vi "Post-Processing VI.vi"() -> ()   [LabVIEW 2014]
uses:
  ATS-VI/ATS_ctl/ExtTrigRange.ctl
  ATS-VI/ATS_ctl/Coupling.ctl
  ATS-VI/ATS_ctl/ExtTrigger.ctl
  ATS-VI/ATS_ctl/TriggerEngine.ctl
  ATS-VI/ATS_ctl/TriggerOperation.ctl
  ATS-VI/ATS_ctl/Trigger.ctl
  ATS-VI/ATS_ctl/Bandwidth.ctl
  ATS-VI/ATS_ctl/Impedance.ctl
  ATS-VI/ATS_ctl/Range.ctl
  ATS-VI/ATS_ctl/InputCtrl.ctl
  ATS-VI/ATS_ctl/ClockEdge.ctl
  ATS-VI/ATS_ctl/ClockRate.ctl
  ATS-VI/ATS_ctl/ClockSource.ctl
  ATS-VI/ATS_ctl/Clock.ctl
  ATS-VI/ATS_ctl/Record.ctl
  ATS-VI/ATS_ctl/ATS_Global.ctl
  Classes/Galvo/Scanning Cluster.ctl
  Classes/Galvo/Galvo.lvclass
  Type Defs/OCT Imaging Parameters Cluster.ctl
  <vilib>/Analysis/NI_AALBase.lvlib
  Type Defs/Imaging Parameters.ctl
  Type Defs/Datalog Format abm.ctl
panel:
  out "No. B-scans":i32=60
  out "system params":T1={"Points Per A-Scan"=0, "A-Scans per B-Scan"=0, "Voltage Range"=4.0, "Card Resolution (bits)"=16}
  in  "Input Parameters":T1={"Points Per A-Scan"=0, "A-Scans per B-Scan"=0, "Voltage Range"=4.0, "Card Resolution (bits)"=16}
  in  "Tab Control":enum32{"Aligned image"}(tab)
  out "Intensity Graph":u8[][](graph)
  in  "Create 3D Data":bool=TRUE
  in  "Max":dbl format="%0.2f"
  in  "Min":dbl format="%0.2f"
  out "Binary File Handle":refnum<file>
  out "En Face":dbl[][](graph)
  out "error out":errorcluster
  out "B-Scan Averaged Across A-Scans":dbl[][](array[numeric])
  in  "En Face Upper Depth":i32=60
  in  "En Face Lower Depth":i32=300
  in  "Cluster":T2={"Imaging Cluster"={"Gain"=6.10352e-05, "Bias"=2.0, "Points Per A-Scan"=-20, "A-Scans per B-Scan"=-20, "Max"=-20.0, "Min"=-20.0}, "OCT Data"=[], "Clock Data"=[]}
  in  "Save B-scans to bmp":bool
  in  "Slide":i32(slide) scale=-1.0..511.0
  in  "Save Image":bool
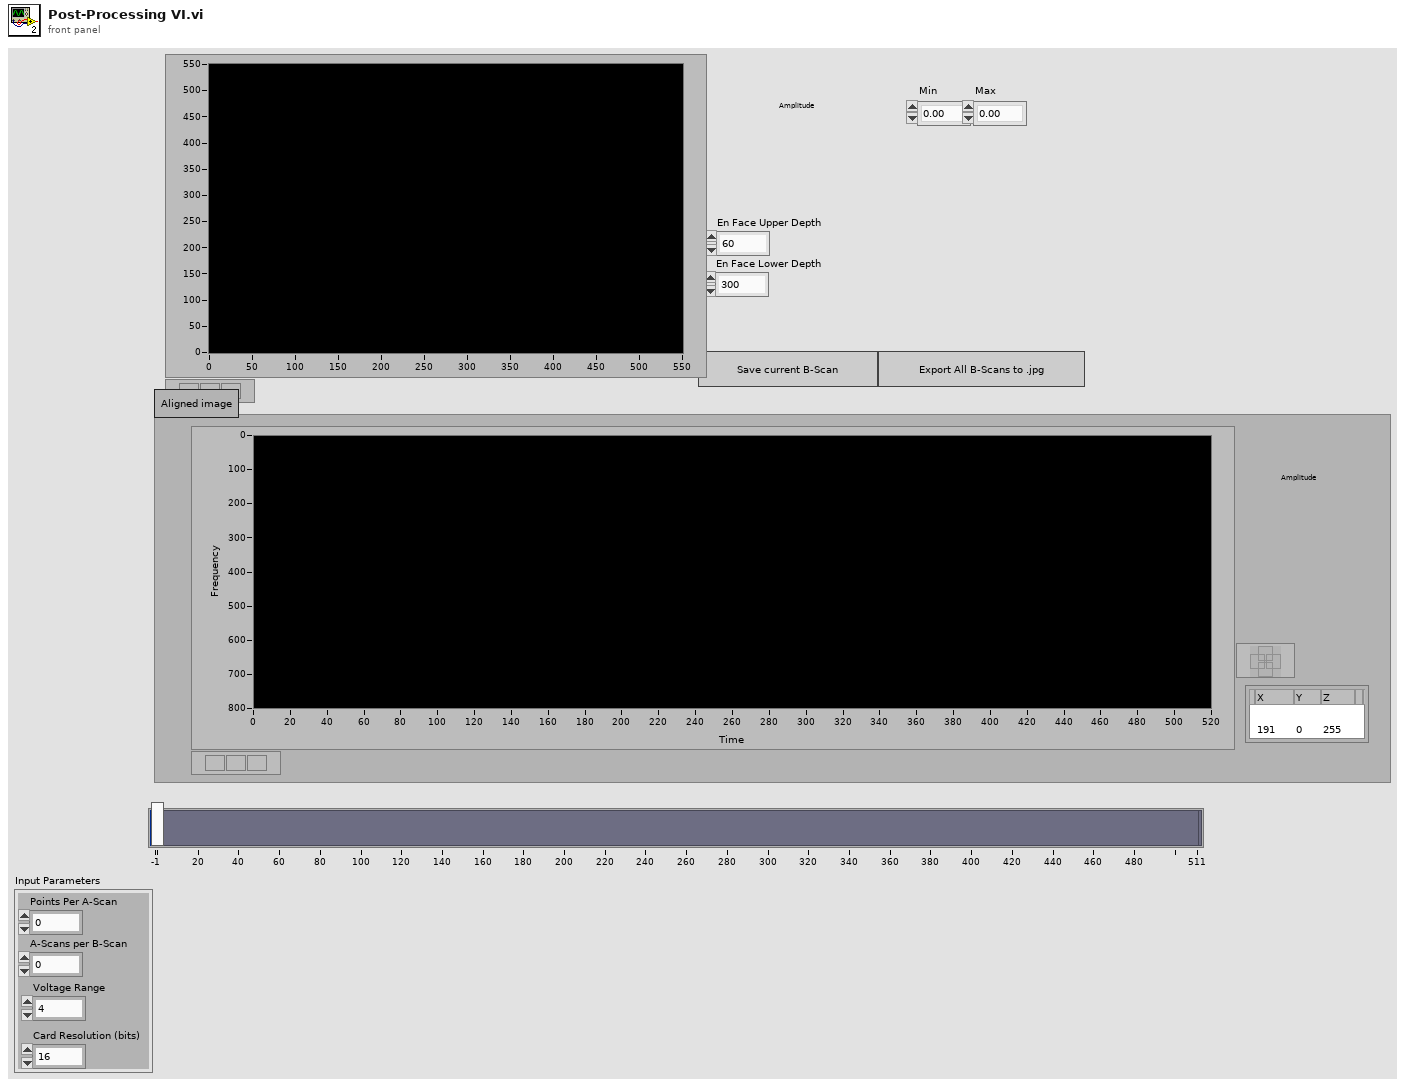
[diagram p1: front panel]
types:
  T1 = typedef "OCT Imaging Parameters Cluster.ctl" = cluster{"Points Per A-Scan":i32, "A-Scans per B-Scan":i32, "Voltage Range":sgl, "Card Resolution (bits)":u16}
  T2 = typedef "Datalog Format abm.ctl" = cluster{"Imaging Cluster":T3, "OCT Data":u16[], "Clock Data":u16[]}
  T3 = typedef "Imaging Parameters.ctl" = cluster{"Gain":sgl, "Bias":sgl, "Points Per A-Scan":i32, "A-Scans per B-Scan":i32, "Max":sgl, "Min":sgl}
  T4 = typedef "Galvo.lvclass/Scanning Cluster.ctl" = cluster{"Fast Axis Offset":sgl, "Slow Axis Offset":sgl, "Slow Axis Amp":sgl, "Fast Axis Amp":sgl, "B-scans (rings)":u32, "A(cluster)/B":u32, "Scan Pattern":enum16{"Raster"}}
  T5 = typedef "ATS_Global.ctl" = cluster{"Record":T6, "Clock":T7, "Input A":T11, "Input B":T11, "Trigger":T16}
  T6 = typedef "Record.ctl" = cluster{"Count":u32, "Presize":u32, "Length":u32}
  T7 = typedef "Clock.ctl" = cluster{"ClckSource":T8, "ClckRate":T9, "ClckEdge":T10, "Decimation":u32}
  T8 = typedef "ClockSource.ctl" = enum16{"Internal", "External", "Medium Ext.", "Slow Ext.", "Ext. AC", "Ext. DC", "Ext. (PLL)"}
  T9 = typedef "ClockRate.ctl" = u32
  T10 = typedef "ClockEdge.ctl" = u16
  T11 = typedef "InputCtrl.ctl" = cluster{"Coupling":T12, "Range":T13, "Impedance":T14, "Bandwidth":T15}
  T12 = typedef "Coupling.ctl" = enum16{"AC", "DC"}
  T13 = typedef "Range.ctl" = u32
  T14 = typedef "Impedance.ctl" = enum16{"1M ohms", "50 ohms"}
  T15 = typedef "Bandwidth.ctl" = enum16{"Full Bandwidth", "Reduce Bandwidth"}
  T16 = typedef "Trigger.ctl" = cluster{"TrigOperation":T17, "Timeout (s)":dbl, "Trig. Delay":u32, "Engine X":T18, "Engine Y":T18, "ExtTrigControl":T19}
  T17 = typedef "TriggerOperation.ctl" = enum16{"Only X", "Only Y", "X or Y", "X and Y", "X xor Y", "X and not Y", "not X and Y"}
  T18 = typedef "TriggerEngine.ctl" = cluster{"Source":enum32{"Chan_A", "Chan_B", "External", "Disable"}, "Slope":enum32{"Positive", "Negative"}, "Level":u32}
  T19 = typedef "ExtTrigger.ctl" = cluster{"Coupling":T12, "Range":T20}
  T20 = typedef "ExtTrigRange.ctl" = enum16{"1 V", "5 V", "TTL"}
  T21 = typedef "imagedata.ctl" = cluster{"image type":i32, "image depth":i32, "image":u8[], "mask":u8[], "colors":u32[], "Rectangle":cluster{"left":i16, "top":i16, "right":i16, "bottom":i16}}
  T22 = cluster{"X Values":dbl[], "Histogram: h(x)":i32[]}
  T23 = typedef "LVRangeTypeDef.ctl" = cluster{"Minimum":dbl, "Maximum":dbl, "Increment":dbl, "Minor Increment":dbl, "Start":dbl}
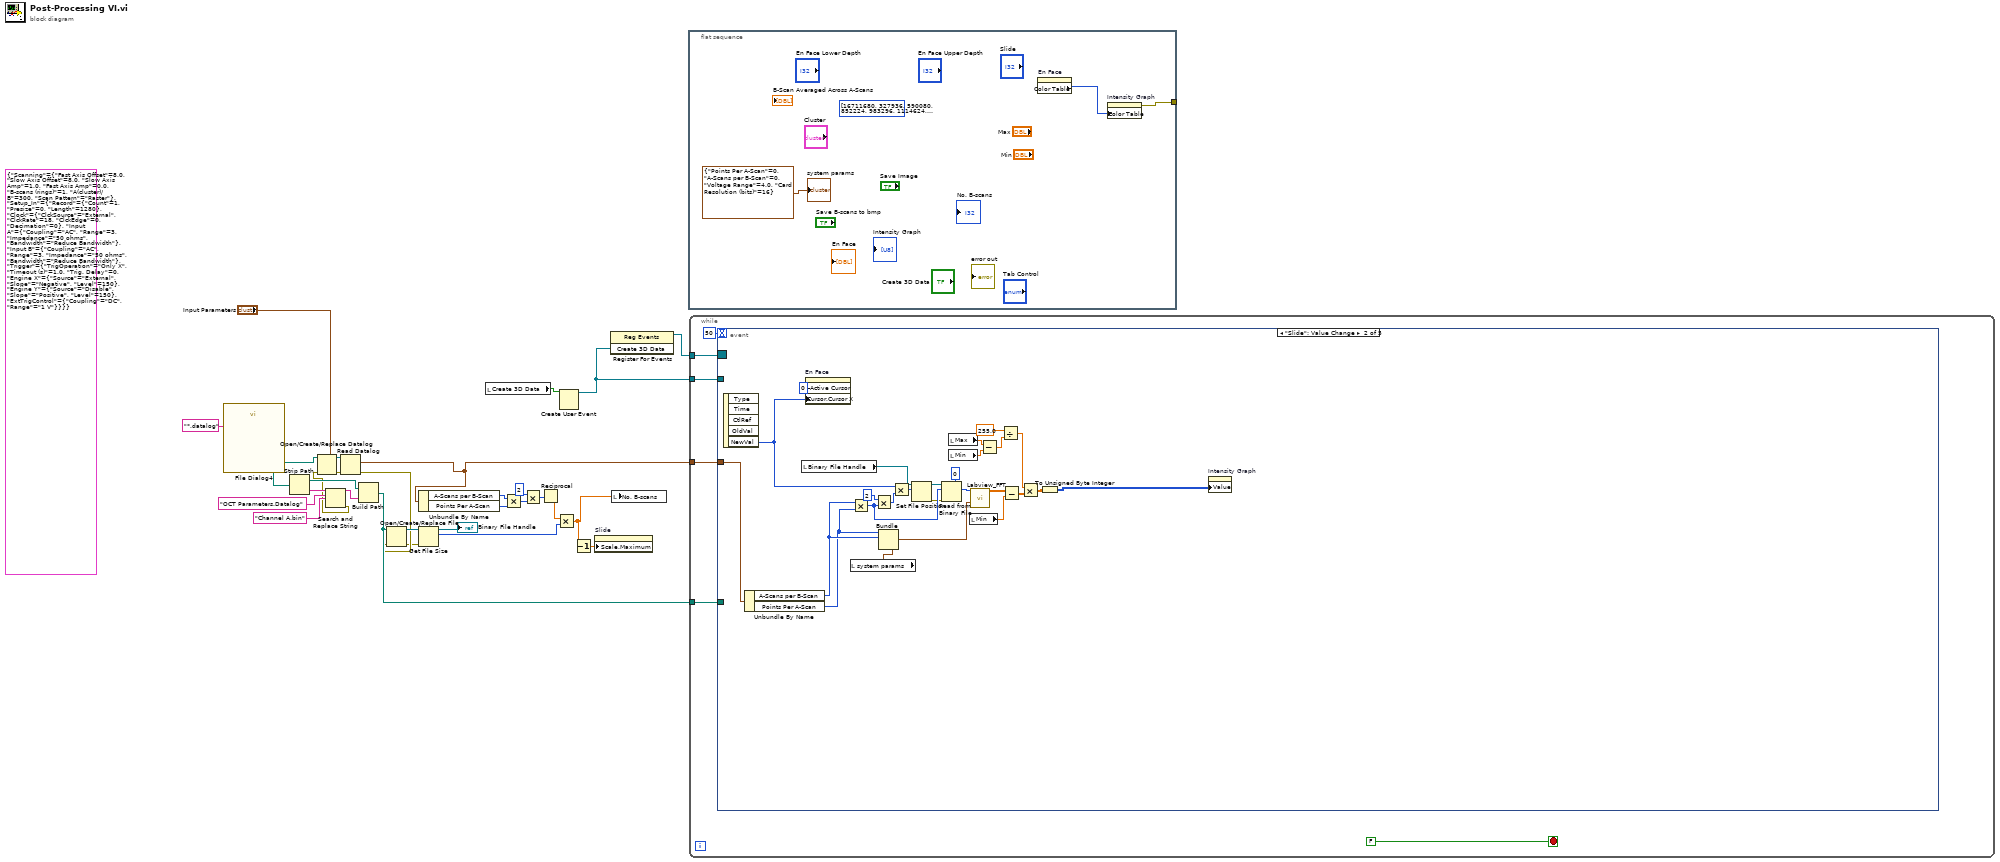
[diagram p0: block diagram]
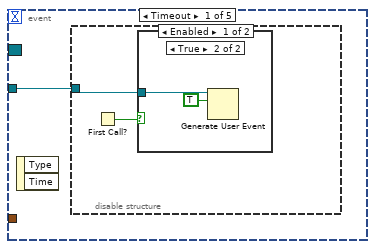
[diagram p2: hidden frame]
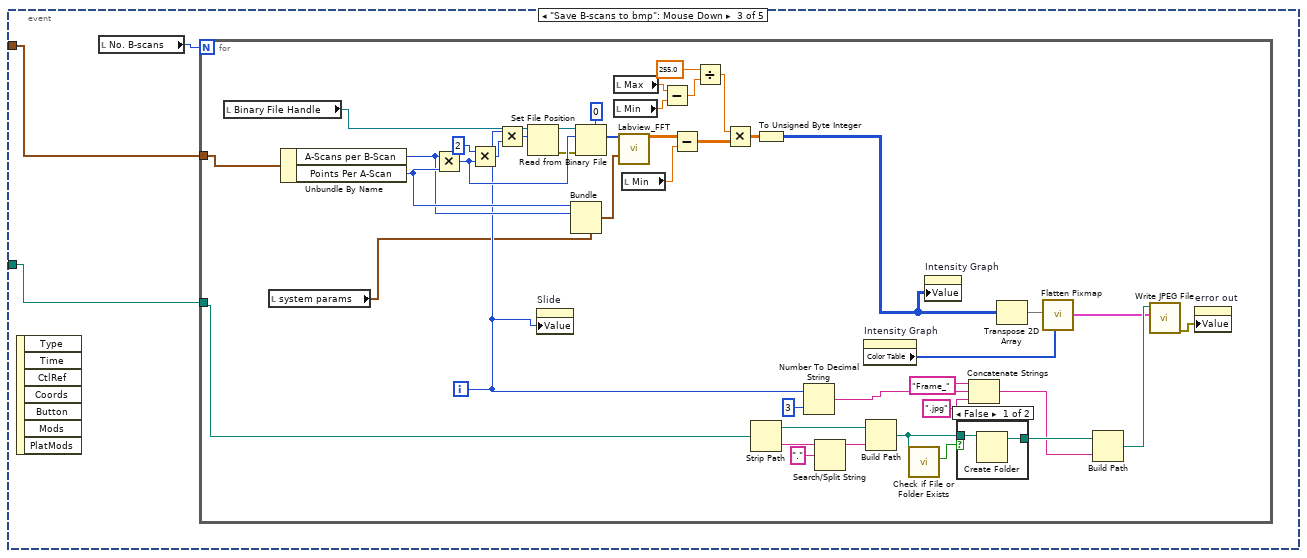
[diagram p5: hidden frame]
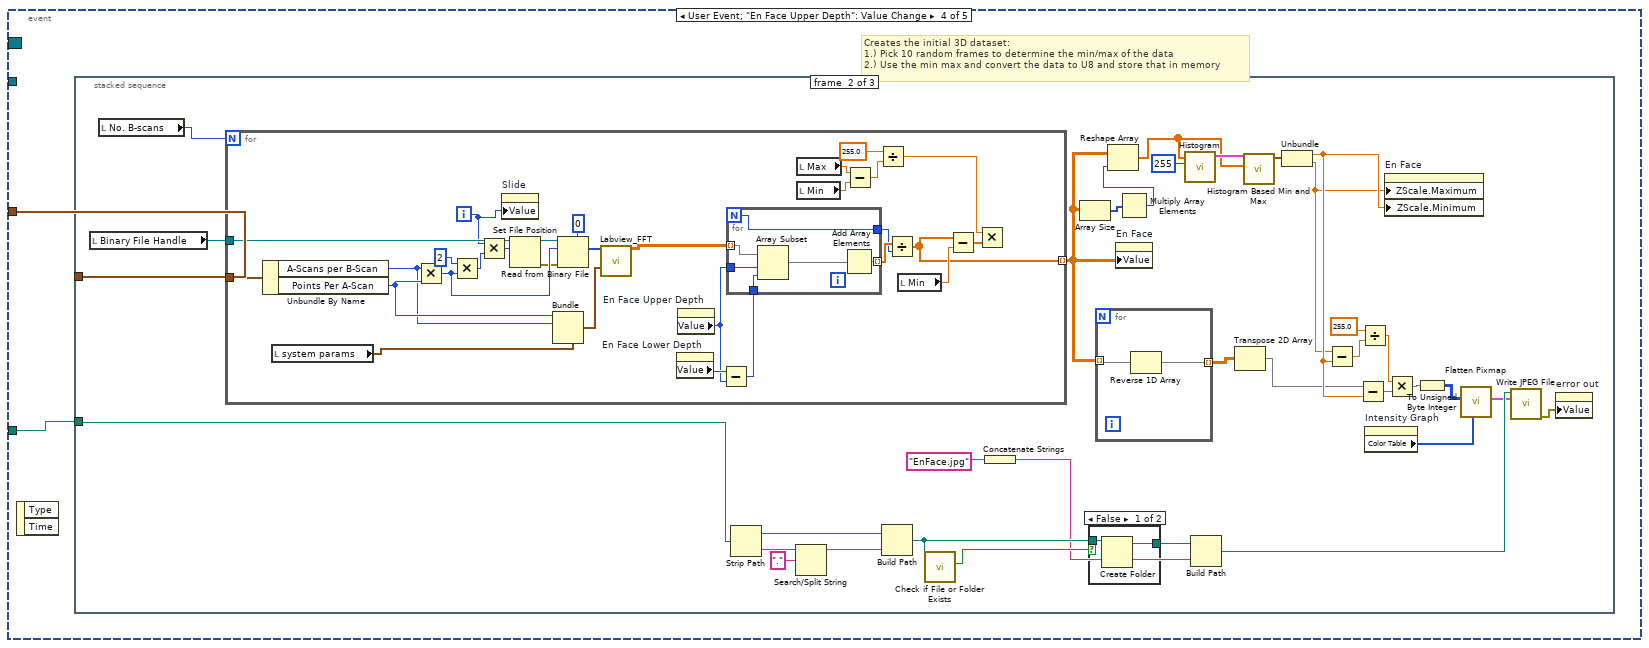
[diagram p7: hidden frame]
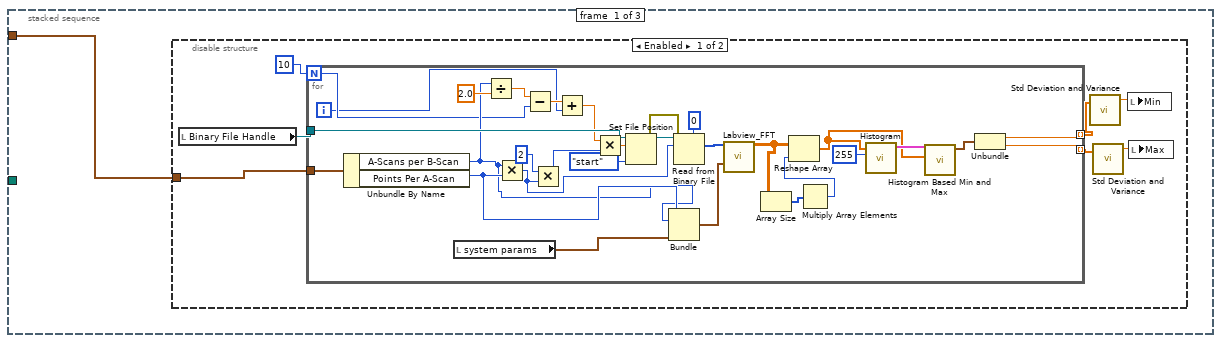
[diagram p8: hidden frame]
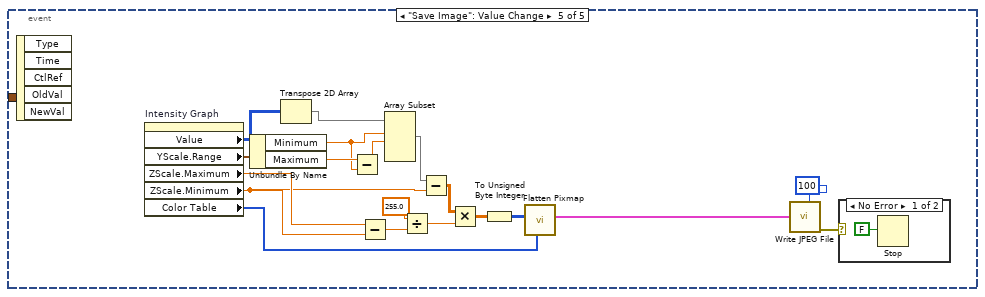
[diagram p12: hidden frame]
diagram:
  (unwired) cluster{"Scanning":T4, "Setup_In":T5} {"Scanning"={"Fast Axis Offset"=8.0, "Slow Axis Offset"=8.0, "Slow Axis Amp"=1.0, "Fast Axis Amp"=0.0, "B-scans (rings)"=1, "A(cluster)/B"=300, "Scan Pattern"=enum."Raster"}, "Setup_In"={"Record"={"Count"=1, "Presize"=0, "Length"=1280}, "Clock"={"ClckSource"=enum."External", "ClckRate"=18, "ClckEdge"=0, "Decimation"=0}, "Input A"={"Coupling"=enum."AC", "Range"=3, "Impedance"=enum."50 ohms", "Bandwidth"=enum."Reduce Bandwidth"}, "Input B"={"Coupling"=enum."AC", "Range"=3, "Impedance"=enum."50 ohms", "Bandwidth"=enum."Reduce Bandwidth"}, "Trigger"={"TrigOperation"=enum."Only X", "Timeout (s)"=1.0, "Trig. Delay"=0, "Engine X"={"Source"=enum."External", "Slope"=enum."Negative", "Level"=150}, "Engine Y"={"Source"=enum."Disable", "Slope"=enum."Positive", "Level"=150}, "ExtTrigControl"={"Coupling"=enum."DC", "Range"=enum."1 V"}}}} ("Sampling Info")
  n1 = call "File Dialog4"("pattern (all files)"="*.datalog") -> ("selected path"=w25:path)  [unwired: 11 in, 3 out]
  n2 = Strip Path(path=w25) -> (stripped path=w21:path, name=w28:string)
  n3 = Search and Replace String(input string=w28, search string="OCT Parameters.Datalog" ("pattern (all files)"), replace string="Channel A.bin" ("pattern (all files)")) -> (result string=w22:string, error out=w6:errorcluster)  [unwired: 5 in, 2 out]
  n4 = Open/Create/Replace Datalog(5:"Input Parameters", 8:w6, 11:w25) -> (0:w23:errorcluster, 3:w24:refnum<k1>)  [unwired: 3 in, 1 out]
  n5 = Read Datalog(4:w23, 7:w24) -> (0:w2:errorcluster, 2:w3:T1)  [unwired: 1 in, 1 out]
  n6 = Build Path(base path=w21, name or relative path=w22) -> (appended path=w12:path)
  n7 = Open/Create/Replace File(file path (use dialog)=w12, error in=w2) -> (refnum out=w20:refnum<file>, error out=w1:errorcluster)  [unwired: 4 in, 1 out]
  n8 = Unbundle By Name(w3) -> ("A-Scans per B-Scan"=w19:i32, "Points Per A-Scan"=w18:i32)
  n9 = Get File Size(file=w20, error in=w1) -> (refnum out=→"Binary File Handle":refnum<file>, size (in bytes)=w14:i64)  [unwired: 1 out]
  n10 = local read "Create 3D Data"() -> (w9:bool)
  n11 = Multiply(x=w19, y=w18) -> (x*y=w17:i32)
  n12 = Multiply(x=u32 2 ("y"), y=w17) -> (x*y=w15:u32)
  n13 = Reciprocal(x=w15) -> (1/x=w13:dbl)
  n14 = Multiply(x=w13, y=w14) -> (x*y=w5:dbl)
  n15 = Create User Event(user event datatype=w9) -> (user event=w8:refnum<user-event>)  [unwired: 1 in, 1 out]
  n16 = Decrement(x=w5) -> (x-1=w4:dbl)
  n17 = property on="Slide" class="Slide (strict)"("Scale.Maximum"=w4) -> ()  [unwired: 2 in, 2 out]
  n18 = register-events(w8) -> (reference out=w11:refnum<event-registration>)  [unwired: 2 in, 1 out]
  n19 = local write "No. B-scans"(w5) -> ()
  n20 = flat-sequence {
    tunnel: [w32] -> _
    frame #0 {
      (unwired) u32[] [16711680, 327936, 590080, 852224, 983296, 1114624, 1180160, 1311232, 1442304, 1573632, 1704704, 1770240, 1901312, 1966848, 2098176, 2163712, 2294784, 2491392, 2557184, 2688256, 2753792, 2884864, 2950656, 3081728, 3147264, 3344129, 3475457, 3540993, 3672321, 3738113, 3869185, 3934977, 4066305, 4197633, 4328961, 4394497, 4460289, 4591617, 4657409, 4788481, 4854273, 4985601, 5116929, 5248257, 5314049, 5379841, 5511169, 5576961, 5708033, 5773825, 5905153, 6036482, 6167810, 6233346, 6299138, 6430466, 6496258, 6562050, 6693634, 6759426, 6890754, 7022082, 7087874, 7153666, 7284994, 7350786, 7482114, 7547906, 7613698, 7745026, 7876354, 8007682, 8073474, 8139522, 8205314, 8336642, 8467970, 8533763, 8599555, 8665347, 8731139, 8862467, 8993795, 9059587, 9125380, 9191428, 9257220, 9388548, 9454340, 9520132, 9585924, 9717253, 9848837, 9914629, 9980165, 10045957, 10177541, 10243334, 10309126, 10375174, 10440966, 10572294, 10703623, 10769416, 10835208, 10901256, 10967049, 11033097, 11033609, 11099401, 11165450, 11231242, 11231754, 11297547, 11363339, 11429131, 11495180, 11495692, 11561740, 11693069, 11758861, 11759373, 11825165, 11891214, 11957006, 12022799, 12023311, 12089103, 12220944, 12286736, 12286736, 12352529, 12418577, 12484370, 12550162, 12615954, 12681747, 12747796, 12813588, 12813845, 12879894, 12945686, 13077015, 13142808, 13143064, 13208856, 13274905, 13340697, 13340953, 13472282, 13538075, 13604379, 13670172, 13735964, 13801757, 13867550, 13933343, 13999392, 13999648, 14065441, 14131234, 14197027, 14197541, 14263334, 14329383, 14395176, 14460969, 14592553, 14658346, 14724139, 14789932, 14790189, 14856238, 14922287, 14988080, 15053873, 15054130, 15119923, 15185972, 15251765, 15317559, 15383353, 15449146, 15449660, 15515454, 15515968, 15516226, 15582021, 15582278, 15582536, 15648587, 15648844, 15714639, 15714897, 15715155, 15780949, 15781463, 15847256, 15847770, 15848028, 15913823, 15914081, 15979875, 15980133, 15980391, 16046441, 16046444, 16046703, 16046705, 16112500, 16113015, 16113274, 16113277, 16179072, 16179330, 16179588, 16245384, 16245387, 16245389, 16245648, 16311443, 16376982, 16377241, 16377499, 16443294, 16443553, 16443555, 16443815, 16509866, 16510124, 16510127, 16575923, 16575924, 16576182, 16576441, 16576443, 16576702, 16576705, 16576963, 16577222, 16577224, 16577482, 16577485, 16577743, 16577745, 16578004, 16578262, 16578264, 16578523, 16578782, 16579040, 16579299, 16579301, 16579303, 16579562, 16579821] ("Color Table")
      n21 = property on="En Face" class="IntGraph (strict)"() -> ("Color Table"=w30:u32[])  [unwired: 2 in, 2 out]
      n22 = property on="Intensity Graph" class="IntGraph (strict)"("Color Table"=w30) -> (error out=w32:errorcluster)  [unwired: 2 in, 1 out]
      "system params" <- T1 {"Points Per A-Scan"=0, "A-Scans per B-Scan"=0, "Voltage Range"=4.0, "Card Resolution (bits)"=16} ("Input Parameters")
    }
  }
  n23 = while {
    tunnel: w3 -> [w36]
    tunnel: w12 -> [w35]
    tunnel: w11 -> [w34]
    tunnel: w8 -> [w33]
    stop <- FALSE stop-if-true
    n24 = event shown="[1] \"Slide\": Value Change" {
      selector: w34 -> [_ _ _ _ _]
      dyn-events: _ -> [_ _ _ _ _]
      timeout: 50 -> [_ _ _ _ _]
      tunnel: w36 -> [_ w68 w72 w120 _]
      tunnel: w35 -> [_ _ w71 w119 _]
      tunnel: w33 -> [w39 _ _ _ _]
      event Timeout {
        n25 = event-data() -> ()  [unwired: 1 in, 2 out]
        n26 = disable-structure shown="Enabled" {
          disable-tunnel: w39 -> [w40 _]
          frame Enabled {
            n27 = First Call?() -> (First Call?: T/F=w41:bool)
            n28 = case shown="True" w41 {
              tunnel: w40 -> [_ w43]
              frame False {
              }
              frame True {
                n29 = Generate User Event(user event=w43, event data cluster=TRUE ("event data")) -> ()  [unwired: 2 in, 2 out]
              }
            }
          }
          frame Disabled {
          }
        }
      }
      event "Slide": Value Change {
        n30 = event-data() -> ("NewVal"=w57:i32)  [unwired: 1 in, 4 out]
        n31 = Unbundle By Name(w68) -> ("A-Scans per B-Scan"=w58:i32, "Points Per A-Scan"=w44:i32)
        n32 = local read "Binary File Handle"() -> (w48:refnum<file>)
        n33 = property on="En Face" class="IntGraph (strict)"("Active Cursor"=u32 0, "Cursor.Cursor X"=w57) -> ()  [unwired: 2 in, 2 out]
        n34 = local read "system params"() -> (w47:T1)
        n35 = Multiply(x=w58, y=w44) -> (x*y=w61:i32)
        n36 = Multiply(x=u32 2 ("y"), y=w61) -> (x*y=w63:u32)
        n37 = Bundle(cluster=w47, "Points Per A-Scan"=w44, "A-Scans per B-Scan"=w58) -> (w59:T1)  [unwired: 2 in]
        n38 = Multiply(x=w57, y=w63) -> (x*y=w65:u32)
        n39 = Set File Position(offset (in bytes) (0)=w65, refnum=w48) -> (refnum out=w66:refnum<file>, error out=w60:errorcluster)  [unwired: 2 in]
        n40 = Read from Binary File(5:u16 0 ("width (-)"), 8:w60, 10:w61, 11:w66) -> (2:w64:u16[])  [unwired: 2 in, 3 out]
        n41 = local read "Max"() -> (w54:dbl)
        n42 = local read "Min"() -> (w53:dbl)
        n43 = local read "Min"() -> (w56:dbl)
        n44 = call "Labview_FFT.vi"("Channel A"=w64, "Input Parameters"=w59) -> ("Int B-Scan Channel A"=w46:sgl[][])  [unwired: 12 in, 1 out]
        n45 = Subtract(x=w54, y=w53) -> (x-y=w52:dbl)
        n46 = Divide(x=255.0, y=w52) -> (x/y=w50:dbl)
        n47 = Subtract(x=w46, y=w56) -> (x-y=w51:dbl[][])
        n48 = Multiply(x=w50, y=w51) -> (x*y=w49:dbl[][])
        n49 = To Unsigned Byte Integer(number=w49) -> (unsigned 8bit integer=w45:u8[][])
        n50 = property on="Intensity Graph" class="IntGraph (strict)"("Value"=w45) -> ()  [unwired: 2 in, 2 out]
      }
      event "Save B-scans to bmp": Mouse Down {
        n51 = event-data() -> ()  [unwired: 1 in, 7 out]
        n52 = local read "No. B-scans"() -> (w70:i32)
        n53 = for {
          N: w70 -> [_]
          tunnel: w72 -> [w78]
          tunnel: w71 -> [w100]
          i -> [w75]
          n54 = local read "Binary File Handle"() -> (w77:refnum<file>)
          n55 = local read "system params"() -> (w74:T1)
          n56 = Unbundle By Name(w78) -> ("A-Scans per B-Scan"=w79:i32, "Points Per A-Scan"=w80:i32)
          n57 = Multiply(x=w79, y=w80) -> (x*y=w92:i32)
          n58 = Multiply(x=u32 2 ("y"), y=w92) -> (x*y=w94:u32)
          n59 = Multiply(x=w75, y=w94) -> (x*y=w96:u32)
          n60 = Set File Position(offset (in bytes) (0)=w96, refnum=w77) -> (refnum out=w97:refnum<file>, error out=w91:errorcluster)  [unwired: 2 in]
          n61 = property on="Slide" class="Slide (strict)"("Value"=w75) -> ()  [unwired: 2 in, 2 out]
          n62 = Bundle(cluster=w74, "Points Per A-Scan"=w80, "A-Scans per B-Scan"=w79) -> (w82:T1)  [unwired: 2 in]
          n63 = Read from Binary File(5:u16 0 ("width (-)"), 8:w91, 10:w92, 11:w97) -> (2:w95:u16[])  [unwired: 2 in, 3 out]
          n64 = local read "Max"() -> (w88:dbl)
          n65 = local read "Min"() -> (w87:dbl)
          n66 = call "Labview_FFT.vi"("Channel A"=w95, "Input Parameters"=w82) -> ("Int B-Scan Channel A"=w81:sgl[][])  [unwired: 12 in, 1 out]
          n67 = local read "Min"() -> (w90:dbl)
          n68 = Subtract(x=w88, y=w87) -> (x-y=w86:dbl)
          n69 = Subtract(x=w81, y=w90) -> (x-y=w85:dbl[][])
          n70 = Divide(x=255.0, y=w86) -> (x/y=w84:dbl)
          n71 = Multiply(x=w84, y=w85) -> (x*y=w83:dbl[][])
          n72 = Strip Path(path=w100) -> (stripped path=w111:path, name=w113:string)
          n73 = To Unsigned Byte Integer(number=w83) -> (unsigned 8bit integer=w76:u8[][])
          n74 = Number To Decimal String(number=w75, width (-)=i16 3) -> (decimal integer string=w109:string)
          n75 = Search/Split String(string=w113, search string/char (-)=".") -> (substring before match=w112:string)  [unwired: 1 in, 2 out]
          n76 = property on="Intensity Graph" class="IntGraph (strict)"() -> ("Color Table"=w115:u32[])  [unwired: 2 in, 2 out]
          n77 = Build Path(base path=w111, name or relative path=w112) -> (appended path=w103:path)
          n78 = call <vilib>:"Check if File or Folder Exists.vi"("path"=w103) -> ("file or folder exists?"=w102:bool)  [unwired: 8 in, 2 out]
          n79 = property on="Intensity Graph" class="IntGraph (strict)"("Value"=w76) -> ()  [unwired: 2 in, 2 out]
          n80 = case shown="False" w102 {
            tunnel: [w117 w118] -> w106
            tunnel: w103 -> [w116 w118]
            frame False {
              n81 = Create Folder(path (use dialog)=w116) -> (created path=w117:path)  [unwired: 2 in, 2 out]
            }
            frame True {
            }
          }
          n82 = Concatenate Strings("Frame_" ("string"), w109, ".jpg" ("string")) -> (w105:string)
          n83 = Transpose 2D Array(2D array=w76) -> (transposed array=w104:u8[][])
          n84 = call <vilib>:"Flatten Pixmap.vi"("colors"=w115, "8-bit pixmap"=w104) -> ("image data"=w73:T21)  [unwired: 9 in]
          n85 = Build Path(base path=w106, name or relative path=w105) -> (appended path=w101:path)
          n86 = call <vilib>:"Write JPEG File.vi"("image data"=w73, "path to JPEG file"=w101) -> ("error out"=w99:errorcluster)  [unwired: 8 in, 1 out]
          n87 = property on="error out" class="Clust (strict)"("Value"=w99) -> ()  [unwired: 2 in, 2 out]
        }
      }
      event User Event; "En Face Upper Depth": Value Change {
        # "Creates the initial 3D dataset:\n1.) Pick 10 random frames to determine the min/max of the data\n2.) Use the min max and convert the data to U8 and store that in memory"
        n88 = event-data() -> ()  [unwired: 1 in, 2 out]
        n89 = stacked-sequence {
          tunnel: w120 -> [w121 w191 _]
          tunnel: w119 -> [_ w177 _]
          frame #0 {
            n90 = disable-structure shown="Enabled" {
              disable-tunnel: w121 -> [w126 _]
              frame Enabled {
                n91 = local read "Binary File Handle"() -> (w128:refnum<file>)
                n92 = for {
                  N: 10 -> [w137]
                  tunnel: w126 -> [w154]
                  tunnel: w128 -> [w153]
                  tunnel: [w142] -> w125 mode=indexing
                  tunnel: [w141] -> w124 mode=indexing
                  i -> [w135]
                  n93 = Unbundle By Name(w154) -> ("A-Scans per B-Scan"=w139:i32, "Points Per A-Scan"=w148:i32)
                  n94 = local read "system params"() -> (w147:T1)
                  n95 = Divide(x=w139, y=2.0) -> (x/y=w138:dbl)
                  n96 = Multiply(x=w139, y=w148) -> (x*y=w133:i32)
                  n97 = Subtract(x=w138, y=w137) -> (x-y=w136:dbl)
                  n98 = Multiply(x=u32 2 ("y"), y=w133) -> (x*y=w152:u32)
                  n99 = Add(x=w136, y=w135) -> (x+y=w134:dbl)
                  n100 = Multiply(x=w134, y=w152) -> (x*y=w156:dbl)
                  n101 = Set File Position(offset (in bytes) (0)=w156, refnum=w153, from (0:start)=enum16{"start", "end", "current"}."start") -> (refnum out=w157:refnum<file>, error out=w150:errorcluster)  [unwired: 1 in]
                  n102 = Bundle(cluster=w147, "Points Per A-Scan"=w148, "A-Scans per B-Scan"=w139) -> (w149:T1)  [unwired: 2 in]
                  n103 = Read from Binary File(5:u16 0 ("width (-)"), 8:w150, 10:w133, 11:w157) -> (2:w155:u16[])  [unwired: 2 in, 3 out]
                  n104 = call "Labview_FFT.vi"("Channel A"=w155, "Input Parameters"=w149) -> ("Int B-Scan Channel A"=w132:sgl[][])  [unwired: 12 in, 1 out]
                  n105 = Array Size(array=w132) -> (size(s)=w131:i32[])
                  n106 = Multiply Array Elements(1:w131) -> (0:w130:i32)
                  n107 = Reshape Array(w132, w130) -> (w144:sgl[])
                  n108 = call <vilib>:"Histogram.vi"("intervals"=255, "X"=w144) -> ("Histogram Graph"=w145:T22)  [unwired: 6 in, 3 out]
                  n109 = call "Histogram Based Min and Max.vi"("Data to Histogram"=w144, "Histogram Graph"=w145) -> ("Histogram Properties"=w143:cluster{"Min":sgl, "Max":sgl})  [unwired: 9 in]
                  n110 = Unbundle(w143) -> ("Min"=w142:sgl, "Max"=w141:sgl)
                }
                n111 = call <vilib>:"Std Deviation and Variance.vi"("X"=w125) -> ("mean"=w123:dbl)  [unwired: 1 in, 2 out]
                n112 = call <vilib>:"Std Deviation and Variance.vi"("X"=w124) -> ("mean"=w122:dbl)  [unwired: 1 in, 2 out]
                n113 = local write "Min"(w123) -> ()
                n114 = local write "Max"(w122) -> ()
              }
              frame Disabled {
              }
            }
          }
          frame #1 {
            n115 = local read "Binary File Handle"() -> (w192:refnum<file>)
            n116 = local read "No. B-scans"() -> (w176:i32)
            n117 = for {
              N: w176 -> [_]
              tunnel: w191 -> [w222]
              tunnel: w192 -> [w221]
              tunnel: [w198] -> w161 mode=indexing
              i -> [w209]
              n118 = Unbundle By Name(w222) -> ("A-Scans per B-Scan"=w214:i32, "Points Per A-Scan"=w215:i32)
              n119 = local read "system params"() -> (w210:T1)
              n120 = Multiply(x=w214, y=w215) -> (x*y=w218:i32)
              n121 = Multiply(x=u32 2 ("y"), y=w218) -> (x*y=w220:u32)
              n122 = Multiply(x=w209, y=w220) -> (x*y=w224:u32)
              n123 = property on="Slide" class="Slide (strict)"("Value"=w209) -> ()  [unwired: 2 in, 2 out]
              n124 = Set File Position(offset (in bytes) (0)=w224, refnum=w221) -> (refnum out=w225:refnum<file>, error out=w217:errorcluster)  [unwired: 2 in]
              n125 = Bundle(cluster=w210, "Points Per A-Scan"=w215, "A-Scans per B-Scan"=w214) -> (w216:T1)  [unwired: 2 in]
              n126 = Read from Binary File(5:u16 0 ("width (-)"), 8:w217, 10:w218, 11:w225) -> (2:w223:u16[])  [unwired: 2 in, 3 out]
              n127 = call "Labview_FFT.vi"("Channel A"=w223, "Input Parameters"=w216) -> ("Int B-Scan Channel A"=w208:sgl[][])  [unwired: 12 in, 1 out]
              n128 = property on="En Face Lower Depth" class="DigNum (strict)"() -> ("Value"=w213:i32)  [unwired: 2 in, 2 out]
              n129 = property on="En Face Upper Depth" class="DigNum (strict)"() -> ("Value"=w212:i32)  [unwired: 2 in, 2 out]
              n130 = Subtract(x=w213, y=w212) -> (x-y=w211:i32)
              n131 = for {
                N -> [w230]
                tunnel: w212 -> [w232]
                tunnel: [w231] -> w207 mode=indexing
                tunnel: [w230] -> w206
                tunnel: w211 -> [w229]
                tunnel: w208 -> [w227] mode=indexing
                n132 = Array Subset(array=w227, index=w232, length=w229) -> (w228:sgl[])
                n133 = Add Array Elements(numeric array=w228) -> (sum=w231:sgl)
              }
              n134 = local read "Max"() -> (w204:dbl)
              n135 = local read "Min"() -> (w203:dbl)
              n136 = Subtract(x=w204, y=w203) -> (x-y=w202:dbl)
              n137 = Divide(x=255.0, y=w202) -> (x/y=w199:dbl)
              n138 = Divide(x=w207, y=w206) -> (x/y=w198:sgl[])
              n139 = local read "Min"() -> (w200:dbl)
              n140 = Subtract(x=w198, y=w200) -> (x-y=w201:dbl[])
              n141 = Multiply(x=w199, y=w201) -> ()  [unwired: 1 out]
            }
            n142 = Strip Path(path=w177) -> (stripped path=w182:path, name=w180:string)
            n143 = Search/Split String(string=w180, search string/char (-)=".") -> (substring before match=w181:string)  [unwired: 1 in, 2 out]
            n144 = Build Path(base path=w182, name or relative path=w181) -> (appended path=w186:path)
            n145 = call <vilib>:"Check if File or Folder Exists.vi"("path"=w186) -> ("file or folder exists?"=w187:bool)  [unwired: 8 in, 2 out]
            n146 = Concatenate Strings("EnFace.jpg" ("string")) -> (w185:string)
            n147 = Array Size(array=w161) -> (size(s)=w171:i32[])
            n148 = case shown="False" w187 {
              tunnel: [w196 w197] -> w184
              tunnel: w186 -> [w195 w197]
              frame False {
                n149 = Create Folder(path (use dialog)=w195) -> (created path=w196:path)  [unwired: 2 in, 2 out]
              }
              frame True {
              }
            }
            n150 = for {
              tunnel: w161 -> [w194] mode=indexing
              tunnel: [w193] -> w160 mode=indexing
              n151 = Reverse 1D Array(array=w194) -> (reversed array=w193:sgl[])
            }
            n152 = property on="En Face" class="IntGraph (strict)"("Value"=w161) -> ()  [unwired: 2 in, 2 out]
            n153 = Multiply Array Elements(1:w171) -> (0:w170:i32)
            n154 = Reshape Array(w161, w170) -> (w173:sgl[])
            n155 = call <vilib>:"Histogram.vi"("intervals"=255, "X"=w173) -> ("Histogram Graph"=w174:T22)  [unwired: 6 in, 3 out]
            n156 = Build Path(base path=w184, name or relative path=w185) -> (appended path=w189:path)
            n157 = Transpose 2D Array(2D array=w160) -> (transposed array=w159:sgl[][])
            n158 = call "Histogram Based Min and Max.vi"("Data to Histogram"=w173, "Histogram Graph"=w174) -> ("Histogram Properties"=w172:cluster{"Min":sgl, "Max":sgl})  [unwired: 9 in]
            n159 = Unbundle(w172) -> ("Min"=w163:sgl, "Max"=w162:sgl)
            n160 = Subtract(x=w162, y=w163) -> (x-y=w169:sgl)
            n161 = Subtract(x=w159, y=w163) -> (x-y=w168:sgl[][])
            n162 = Divide(x=sgl 255.0, y=w169) -> (x/y=w167:sgl)
            n163 = property on="Intensity Graph" class="IntGraph (strict)"() -> ("Color Table"=w178:u32[])  [unwired: 2 in, 2 out]
            n164 = property on="En Face" class="IntGraph (strict)"("ZScale.Maximum"=w162, "ZScale.Minimum"=w163) -> ()  [unwired: 2 in, 2 out]
            n165 = Multiply(x=w167, y=w168) -> (x*y=w166:sgl[][])
            n166 = To Unsigned Byte Integer(number=w166) -> (unsigned 8bit integer=w164:u8[][])
            n167 = call <vilib>:"Flatten Pixmap.vi"("colors"=w178, "8-bit pixmap"=w164) -> ("image data"=w188:T21)  [unwired: 9 in]
            n168 = call <vilib>:"Write JPEG File.vi"("image data"=w188, "path to JPEG file"=w189) -> ("error out"=w190:errorcluster)  [unwired: 8 in, 1 out]
            n169 = property on="error out" class="Clust (strict)"("Value"=w190) -> ()  [unwired: 2 in, 2 out]
          }
          frame #2 {
          }
        }
      }
      event "Save Image": Value Change {
        n170 = event-data() -> ()  [unwired: 1 in, 5 out]
        n171 = property on="Intensity Graph" class="IntGraph (strict)"() -> ("Value"=w233:u8[][], "YScale.Range"=w239:T23, "ZScale.Maximum"=w251:dbl, "ZScale.Minimum"=w250:dbl, "Color Table"=w243:u32[])  [unwired: 2 in, 2 out]
        n172 = Unbundle By Name(w239) -> ("Minimum"=w236:dbl, "Maximum"=w237:dbl)
        n173 = Transpose 2D Array(2D array=w233) -> (transposed array=w234:u8[][])
        n174 = Subtract(x=w237, y=w236) -> (x-y=w235:dbl)
        n175 = Subtract(x=w251, y=w250) -> (x-y=w249:dbl)
        n176 = Array Subset(array=w234, index (row)=w236, length (row)=w235) -> (w238:u8[][])  [unwired: 2 in]
        n177 = Divide(x=255.0, y=w249) -> (x/y=w247:dbl)
        n178 = Subtract(x=w238, y=w250) -> (x-y=w246:dbl[][])
        n179 = Multiply(x=w246, y=w247) -> (x*y=w245:dbl[][])
        n180 = To Unsigned Byte Integer(number=w245) -> (unsigned 8bit integer=w244:u8[][])
        n181 = call <vilib>:"Flatten Pixmap.vi"("colors"=w243, "8-bit pixmap"=w244) -> ("image data"=w242:T21)  [unwired: 9 in]
        n182 = call <vilib>:"Write JPEG File.vi"("quality (80)"=100, "image data"=w242) -> ("error out"=w240:errorcluster)  [unwired: 8 in, 1 out]
        n183 = case shown="No Error" w240 {
          frame No Error {
            n184 = Stop(stop? (T)=FALSE) -> ()
          }
          frame Error {
          }
        }
      }
    }
  }
